vi "Action Update Set Point.vi"(8 "error in (no error)":errorcluster, 11 "Temperature Set Point":dbl) -> (0 "error out":errorcluster)   [LabVIEW 2018, in "Thermal Chamber Controller_DQMH.lvlib"]
uses:
  Thermal Chamber Controller_DQMH.lvlib
  Thermal Chamber Response Simulator/Thermal Chamber Response Simulator.lvlib
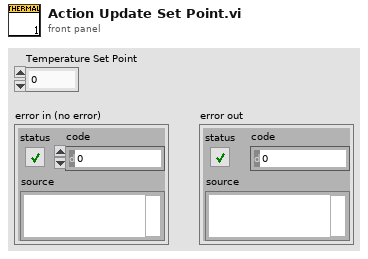
[diagram p1: front panel]
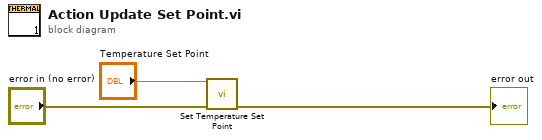
[diagram p0: block diagram]
diagram:
  n1 = call "Set Temperature Set Point.vi"("error in (no error)"="error in (no error)", "Temperature Set Point (deg C)"="Temperature Set Point") -> ("error out"=→"error out":errorcluster)  [unwired: 9 in]
